vi "Main.vi"() -> ()   [LabVIEW 2020, in "ATM Machine.lvlib"]
doc: "This template is for the Queued Message Handler design pattern.\n\nThe Event Handling Loop generates messages based on user interface actions.\n\nThe Message Handling Loop processes messages generated by the Event Handling Loop, or by other messages. The messages are string values, so new messages can be added easily to the Message Cases case structure in the Message Handling Loop. Each message cluster can also provide an optional value for Message Data, which is a variant that can be converted to whatever message-specific data is required."
uses:
  ATM Machine/ATM Machine.lvlib
  Users/khemr/OneDrive/Desktop/Labview Training/CLD/New ATM_KR/ATM Machine/Cluster - Message Cluster.ctl
  ATM Machine/Cluster - ATM Machine Data.ctl
  ATM Machine/Enum - ATM States.ctl
panel:
  in  "Right Menu":T1
  in  "Left Menu":T1
  in  "Enter":bool
  in  "User Input":string
  in  "Right Buttons":T2
  in  "Left Buttons":T2
  in  "Card Simulator":bool
  out "ATM Messages":string
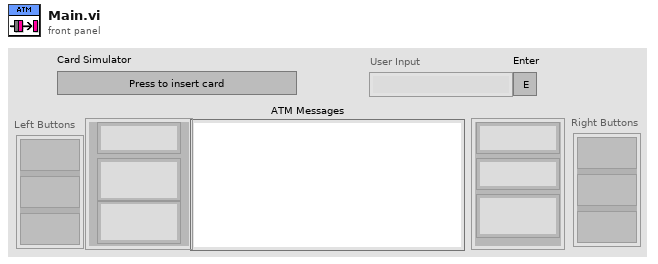
[diagram p1: front panel]
types:
  T1 = cluster{"String":string, "String 2":string, "String 3":string}
  T2 = cluster{"Func Button":bool, "Func Button 2":bool, "Func Button 3":bool}
  T3 = typedef "ATM Machine.lvlib/Cluster - ATM Machine Data.ctl" = cluster{"UI Refs":cluster{"Right Buttons":refnum<vi>, "Left Buttons":refnum<vi>, "User Input":refnum<vi>, "ATM Messages":refnum<vi>, "Left Menu":refnum<vi>, "Right Menu":refnum<vi>, "Enter":refnum<vi>}, "Map":map{string, cluster{"Pin":string, "First Name":string, "Last Name":string, "Balance":dbl}}, "Login Valid?":bool, "Queue Message":refnum<queue>, "State":T4, "User":cluster{"Pin":string, "First Name":string, "Last Name":string, "Balance":dbl, "Login Valid?":bool}, "Main States":cluster{"Message":string, "Data":variant}}
  T4 = typedef "ATM Machine.lvlib/Enum - ATM States.ctl" = enum16{"None", "Deposit", "Withdraw", "Card Inserted", "Balance Inquiry", "Return Card and Terminate", "Fast Cash"}
  T5 = typedef "ATM Machine.lvlib/Cluster - Message Cluster.ctl" = cluster{"Message":string, "Data":variant}
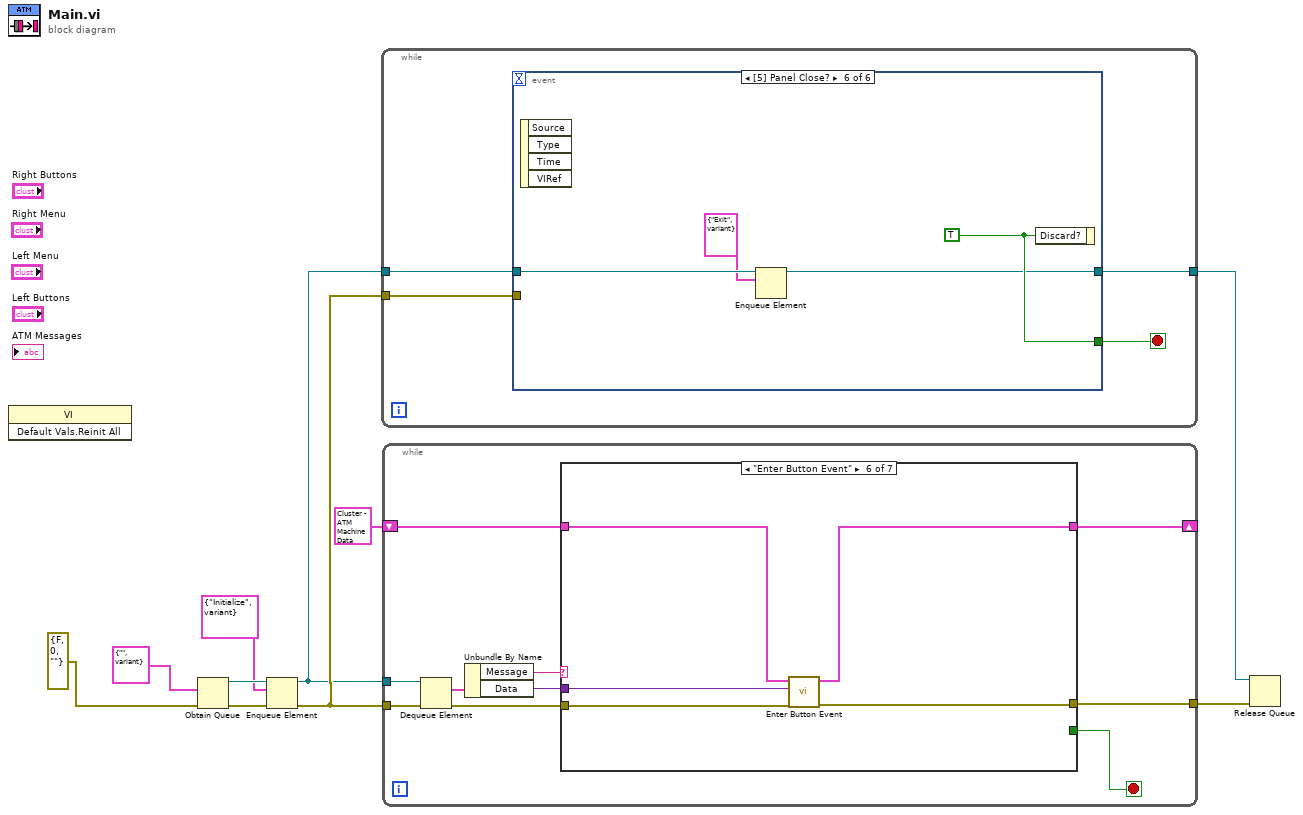
[diagram p0: block diagram]
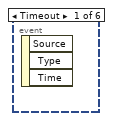
[diagram p2: hidden frame]
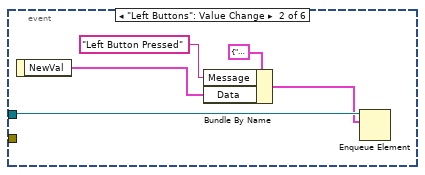
[diagram p3: hidden frame]
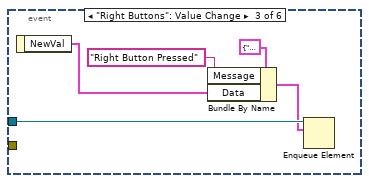
[diagram p4: hidden frame]
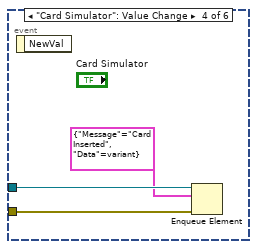
[diagram p5: hidden frame]
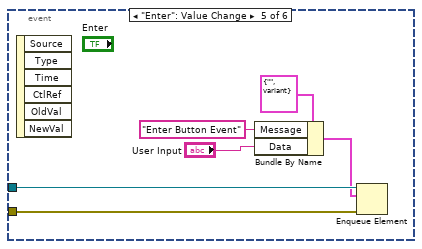
[diagram p6: hidden frame]
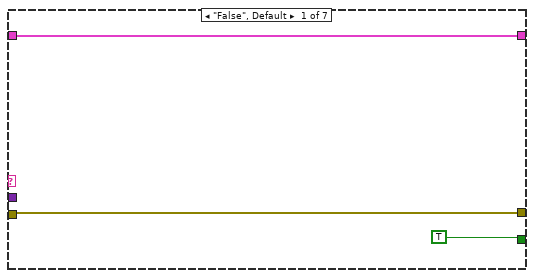
[diagram p7: hidden frame]
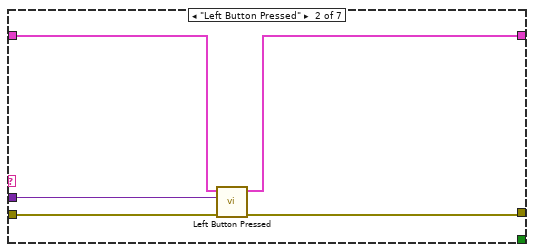
[diagram p8: hidden frame]
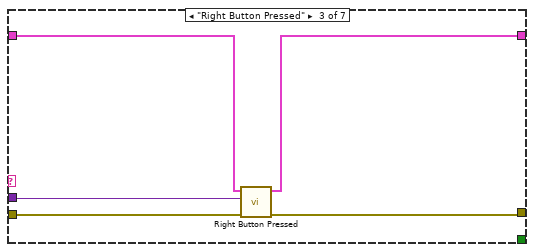
[diagram p9: hidden frame]
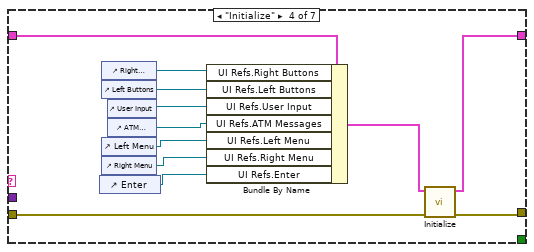
[diagram p10: hidden frame]
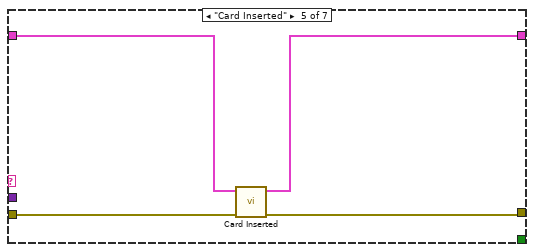
[diagram p11: hidden frame]
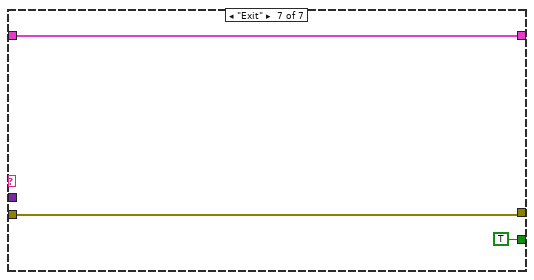
[diagram p12: hidden frame]
diagram:
  n1 = invoke class="VI" method="Default Vals.Reinit All"() -> ()  [unwired: 3 in, 3 out]
  n2 = Obtain Queue(element data type=T5 {"Message"="", "Data"=variant}, error in (no error)=errorcluster {"status"=FALSE, "code"=0, "source"=""} ("error constant")) -> (queue out=w7:refnum<queue>, error out=w8:errorcluster)  [unwired: 3 in, 1 out]
  n3 = Enqueue Element(queue=w7, element=cluster{"Message":string, "Data":variant} {"Message"="Initialize", "Data"=variant}, error in (no error)=w8) -> (queue out=w3:refnum<queue>, error out=w4:errorcluster)  [unwired: 1 in, 1 out]
  n4 = while {
    tunnel: w3 -> [w14]
    tunnel: w4 -> [w13]
    tunnel: [w12] -> w1
    stop <- w11 stop-if-true
    n5 = event shown="[5] Panel Close?" {
      selector: _ -> [_ _ _ _ _ _]
      dyn-events: _ -> [_ _ _ _ _ _]
      timeout: _ -> [_ _ _ _ _ _]
      tunnel: w14 -> [_ w19 w24 w27 w33 w35]
      tunnel: w13 -> [_ _ _ w25 w32 _]
      tunnel: [_ _ _ _ _ w36] -> w12
      tunnel: [_ _ _ _ _ w37] -> w11
      event Timeout {
        n6 = event-data() -> ()  [unwired: 1 in, 3 out]
      }
      event "Left Buttons": Value Change {
        n7 = event-data() -> ("NewVal"=w17:T2)  [unwired: 1 in]
        n8 = Bundle By Name(cluster=cluster{"Message":string, "Data":variant} {"Message"="", "Data"=variant} ("element"), "Message"="Left Button Pressed", "Data"=w17) -> (w15:cluster{"Message":string, "Data":variant})
        n9 = Enqueue Element(queue=w19, element=w15) -> ()  [unwired: 2 in, 3 out]
      }
      event "Right Buttons": Value Change {
        n10 = event-data() -> ("NewVal"=w21:T2)  [unwired: 1 in]
        n11 = Bundle By Name(cluster=cluster{"Message":string, "Data":variant} {"Message"="", "Data"=variant} ("element"), "Message"="Right Button Pressed", "Data"=w21) -> (w20:cluster{"Message":string, "Data":variant})
        n12 = Enqueue Element(queue=w24, element=w20) -> ()  [unwired: 2 in, 3 out]
      }
      event "Card Simulator": Value Change {
        n13 = event-data() -> ()  [unwired: 1 in, 1 out]
        n14 = Enqueue Element(queue=w27, element=cluster{"Message":string, "Data":variant} {"Message"="Card Inserted", "Data"=variant}, error in (no error)=w25) -> ()  [unwired: 1 in, 3 out]
      }
      event "Enter": Value Change {
        n15 = event-data() -> ()  [unwired: 1 in, 6 out]
        n16 = Bundle By Name(cluster=T5 {"Message"="", "Data"=variant} ("element"), "Message"="Enter Button Event", "Data"="User Input") -> (w30:T5)
        n17 = Enqueue Element(queue=w33, element=w30, error in (no error)=w32) -> ()  [unwired: 1 in, 3 out]
      }
      event Panel Close? {
        w37 = TRUE ("Discard?")
        n18 = event-data() -> ()  [unwired: 1 in, 4 out]
        n19 = Enqueue Element(queue=w35, element=T5 {"Message"="Exit", "Data"=variant}) -> (queue out=w36:refnum<queue>)  [unwired: 2 in, 2 out]
        n20 = event-data("Discard?"=w37) -> ()  [unwired: 1 in, 1 out]
      }
    }
  }
  n21 = while {
    tunnel: w3 -> [w47]
    tunnel: w4 -> [w45]
    tunnel: [w44] -> w2
    shift-right: [w39] -> _
    shift-left: T3 {"UI Refs"={"Right Buttons"=refnum, "Left Buttons"=refnum, "User Input"=refnum, "ATM Messages"=refnum, "Left Menu"=refnum, "Right Menu"=refnum, "Enter"=refnum}, "Map"={}, "Login Valid?"=FALSE, "Queue Message"=refnum, "State"=enum."None", "User"={"Pin"="", "First Name"="", "Last Name"="", "Balance"=0.0, "Login Valid?"=FALSE}, "Main States"={"Message"="Initialize", "Data"=variant}} ("Cluster") -> [w40]
    stop <- w42 stop-if-true
    n22 = Dequeue Element(queue=w47, error in (no error)=w45) -> (element=w41:T5, error out=w43:errorcluster)  [unwired: 1 in, 2 out]
    n23 = Unbundle By Name(w41) -> ("Message"=w46:string, "Data"=w38:variant)
    n24 = case shown="\"Enter Button Event\"" w46 {
      tunnel: [w50 w54 w60 w72 w76 w80 w83] -> w44
      tunnel: w43 -> [w50 w53 w59 w71 w75 w81 w83]
      tunnel: [TRUE _ _ _ _ _ TRUE] -> w42
      tunnel: w40 -> [w48 w52 w57 w66 w73 w78 w84]
      tunnel: [w48 w55 w58 w64 w74 w79 w84] -> w39
      tunnel: w38 -> [_ w51 w56 _ _ w77 _]
      frame "False", Default {
      }
      frame "Left Button Pressed" {
        n25 = call "Left Button Pressed.vi"("error in"=w53, "variant"=w51, "ATM Data"=w52) -> ("error out"=w54:errorcluster, "ATM Data Out"=w55:T3)  [unwired: 7 in]
      }
      frame "Right Button Pressed" {
        n26 = call "Right Button Pressed.vi"("error in"=w59, "variant"=w56, "ATM Data"=w57) -> ("error out"=w60:errorcluster, "ATM Data Out"=w58:T3)  [unwired: 7 in]
      }
      frame "Initialize" {
        n27 = control-ref of="Enter"() -> (w61:refnum<vi>)
        n28 = control-ref of="Right Buttons"() -> (w70:refnum<vi>)
        n29 = control-ref of="Left Buttons"() -> (w69:refnum<vi>)
        n30 = control-ref of="Left Menu"() -> (w63:refnum<vi>)
        n31 = control-ref of="Right Menu"() -> (w62:refnum<vi>)
        n32 = control-ref of="User Input"() -> (w68:refnum<vi>)
        n33 = control-ref of="ATM Messages"() -> (w67:refnum<vi>)
        n34 = Bundle By Name(cluster=w66, "UI Refs.Right Buttons"=w70, "UI Refs.Left Buttons"=w69, "UI Refs.User Input"=w68, "UI Refs.ATM Messages"=w67, "UI Refs.Left Menu"=w63, "UI Refs.Right Menu"=w62, "UI Refs.Enter"=w61) -> (w65:T3)
        n35 = call "Initialize.vi"("error in (no error)"=w71, "ATM Data"=w65) -> ("error out"=w72:errorcluster, "ATM Data Out"=w64:T3)  [unwired: 8 in]
      }
      frame "Card Inserted" {
        n36 = call "Card Inserted.vi"("error in"=w75, "ATM Data"=w73) -> ("error out"=w76:errorcluster, "ATM Data Out"=w74:T3)  [unwired: 8 in]
      }
      frame "Enter Button Event" {
        n37 = call "Enter Button Event.vi"("error in (no error)"=w81, "Variant"=w77, "ATM Data"=w78) -> ("error out"=w80:errorcluster, "ATM Data Out"=w79:T3)  [unwired: 7 in]
      }
      frame "Exit" {
      }
    }
  }
  n38 = Release Queue(queue=w1, error in (no error)=w2) -> ()  [unwired: 1 in, 3 out]
